vi "Dig Test.vi"   [LabVIEW 2017, in "Tests.lvlib"]
uses:
  Tests.lvlib
  Dig Target.vi
  src/Toolkit VIs/Toolkit VIs.lvlib
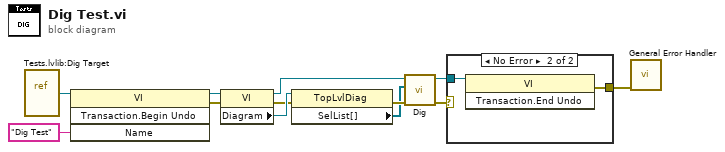
[diagram p0: block diagram]
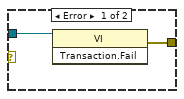
[diagram p2: hidden frame]
diagram:
  n1 = vi-ref "Tests.lvlib:Dig Target.vi"() -> (w6:refnum<vi>)
  n2 = invoke class="VI" method="Transaction.Begin Undo"(reference=w6, "Name"="Dig Test") -> (reference out=w10:refnum<vi>, error out=w8:errorcluster)  [unwired: 2 in, 2 out]
  n3 = property class="VI"(reference=w10, error in=w8) -> (reference out=w5:refnum<vi>, error out=w11:errorcluster, "Diagram"=w12:refnum<vi>)
  n4 = property class="TopLvlDiag"(reference=w12, error in=w11) -> (error out=w7:errorcluster, "SelList[]"=w4:refnum<vi>[])  [unwired: 1 out]
  n5 = call "Dig.vi"("Error In"=w7, "Selection List[]"=w4, "VI In"=w5) -> ("Error Out"=w1:errorcluster, "VI Out"=w3:refnum<vi>)  [unwired: 7 in]
  n6 = case shown="No Error" w1 {
    tunnel: [w14 w16] -> w2
    tunnel: w3 -> [w13 w15]
    frame Error {
      n7 = invoke class="VI" method="Transaction.Fail"(reference=w13) -> (error out=w14:errorcluster)  [unwired: 2 in, 2 out]
    }
    frame No Error {
      n8 = invoke class="VI" method="Transaction.End Undo"(reference=w15) -> (error out=w16:errorcluster)  [unwired: 2 in, 2 out]
    }
  }
  n9 = call <vilib>:"General Error Handler.vi"("error in (no error)"=w2) -> ()  [unwired: 10 in, 5 out]
